vi "Execute.LoadSequences.vi"(8 "error in (no error)":errorcluster, 11 "Cluster":T1={"NIVS.BaseLogPath"=path "", "NIVS.SystemDefinitionFile"=path "", "NIVS.Events"={"SequenceEvent"=refnum, "SystemChangeEvent"=refnum, "WorkspaceEvent"=refnum}, "NIVS.SequenceState"=enum."Idle", "NIVS.GatewayIPAddress"="", "NIVS.DataLogSpecRef"=refnum, "NIVS.DataLogManagerRef"=refnum, "NIVS.LogSessionGUID"="", "NIVS.WorkspaceManager"=refnum, "NIVS.Deployed"=FALSE, "NIVS.ProfileRef"=refnum, "NIVS.ProfileCallback"=refnum, "NIVS.SystemStateRefs"={"CustDatRef"=refnum, "EvtRef"=refnum}, "UI.Abort"=refnum, "UI.Pause"=refnum, "UI.EnableLogging"=refnum, "UI.Start"=refnum, "UI.LogChannels"=refnum, "UI.StartIteration"=refnum, "UI.StartStep"=refnum, "UI.Sequence"=refnum, "UI.PreviewMode"=refnum, "UI.Graph"=refnum, "UI.BaseFileName"=refnum, "UI.Profiles"=refnum, "UI.CurrentStep"=refnum, "UI.CurrentIteration"=refnum, "UI.TotalIterations"=refnum, "Sequence.AbortChannel"="", "Sequence.StepInfoChannel"="", "Sequence.Iterations"=0, "Sequence.IterationInfoChannel"="", "Sequence.#ofColumns"=0, "Events.State"=refnum, "Events.Test Result"=refnum, "Events.Progress"=refnum, "INI.Settings"={"Build Location"=path "C:/Simple Sequence Editor/SequenceRepo", "LoggingLocation"=path ""}}) -> (0 "error out":errorcluster)   [LabVIEW 2013, in "Simple Sequence Tools - Execution.lvlib"]
uses:
  Simple Sequence Tools - Execution.lvlib
  Types/Execuction.StateVariables.ctl
  Types/Execute.UserEventRefs.ctl
  <vilib>/NI Veristand/Execution/Workspace/SystemStateRegEventRef.ctl
  Types/Execution.SequenceState.ctl
  <vilib>/NI Veristand/Execution/DataLogging/DataLoggingSpecification Ref.ctl
  NationalInstruments.VeriStand.ClientAPI
  <vilib>/NI Veristand/Execution/DataLogging/IDataLogging Ref.ctl
  <vilib>/NI Veristand/Execution/Workspace/WorkspaceAPI.ctl
  NationalInstruments.VeriStand.RealTimeSequenceDefinitionApi
  <vilib>/NI Veristand/Execution/Workspace/SystemStateEventRef.ctl
  Shared/Types/INI.Settings
  Shared/Simple Sequence Tools - Shared.lvlib
  <vilib>/NI Veristand/Execution/Workspace/NI_VS Workspace ExecutionAPI.lvlib
  <vilib>/NI Veristand/Execution/DataLogging/NI_VS Data Logging API.lvlib
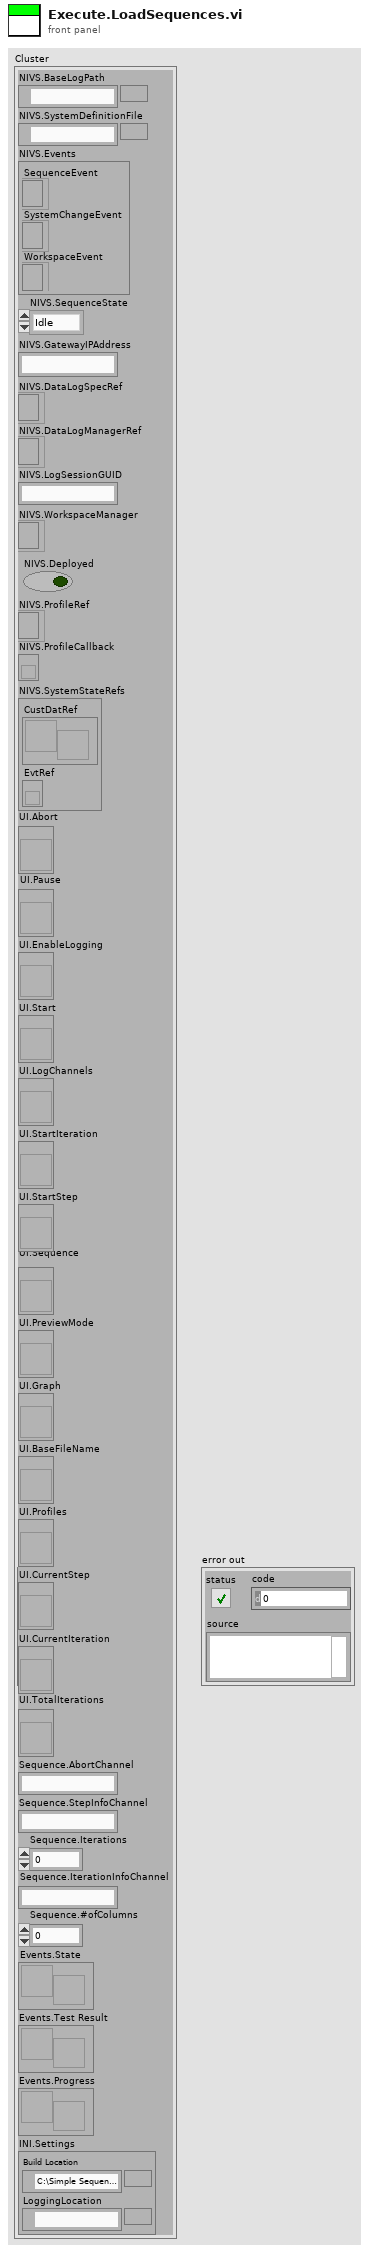
[diagram p1: front panel]
types:
  T1 = typedef "Simple Sequence Tools - Execution.lvlib/Execuction.StateVariables.ctl" = cluster{"NIVS.BaseLogPath":path, "NIVS.SystemDefinitionFile":path, "NIVS.Events":T2, "NIVS.SequenceState":T4, "NIVS.GatewayIPAddress":string, "NIVS.DataLogSpecRef":T5, "NIVS.DataLogManagerRef":T6, "NIVS.LogSessionGUID":string, "NIVS.WorkspaceManager":T7, "NIVS.Deployed":bool, "NIVS.ProfileRef":refnum<k24>, "NIVS.ProfileCallback":refnum<k27>, "NIVS.SystemStateRefs":T8, "UI.Abort":refnum<vi>, "UI.Pause":refnum<vi>, "UI.EnableLogging":refnum<vi>, "UI.Start":refnum<vi>, "UI.LogChannels":refnum<vi>, "UI.StartIteration":refnum<vi>, "UI.StartStep":refnum<vi>, "UI.Sequence":refnum<vi>, "UI.PreviewMode":refnum<vi>, "UI.Graph":refnum<vi>, "UI.BaseFileName":refnum<vi>, "UI.Profiles":refnum<vi>, "UI.CurrentStep":refnum<vi>, "UI.CurrentIteration":refnum<vi>, "UI.TotalIterations":refnum<vi>, "Sequence.AbortChannel":string, "Sequence.StepInfoChannel":string, "Sequence.Iterations":u32, "Sequence.IterationInfoChannel":string, "Sequence.#ofColumns":i32, "Events.State":refnum<user-event>, "Events.Test Result":refnum<user-event>, "Events.Progress":refnum<user-event>, "INI.Settings":T9}
  T2 = typedef "Simple Sequence Tools - Execution.lvlib/Execute.UserEventRefs.ctl" = cluster{"SequenceEvent":refnum<event-registration>, "SystemChangeEvent":T3, "WorkspaceEvent":refnum<event-registration>}
  T3 = typedef "NI_VS Workspace ExecutionAPI.lvlib/SystemStateRegEventRef.ctl" = refnum<event-registration>
  T4 = typedef "Simple Sequence Tools - Execution.lvlib/Execution.SequenceState.ctl" = enum16{"Idle", "Initializing", "Running", "Paused", "Finalizing", "Complete"}
  T5 = typedef "NI_VS Data Logging API.lvlib/DataLoggingSpecification Ref.ctl" = refnum<k24>
  T6 = typedef "NI_VS Data Logging API.lvlib/IDataLogging Ref.ctl" = refnum<k24>
  T7 = typedef "NI_VS Workspace ExecutionAPI.lvlib/WorkspaceAPI.ctl" = refnum<k24>
  T8 = typedef "NI_VS Workspace ExecutionAPI.lvlib/SystemStateEventRef.ctl" = cluster{"CustDatRef":refnum<user-event>, "EvtRef":refnum<k27>}
  T9 = typedef "Simple Sequence Tools - Shared.lvlib/INI.Settings" = cluster{"Build Location":path, "LoggingLocation":path}
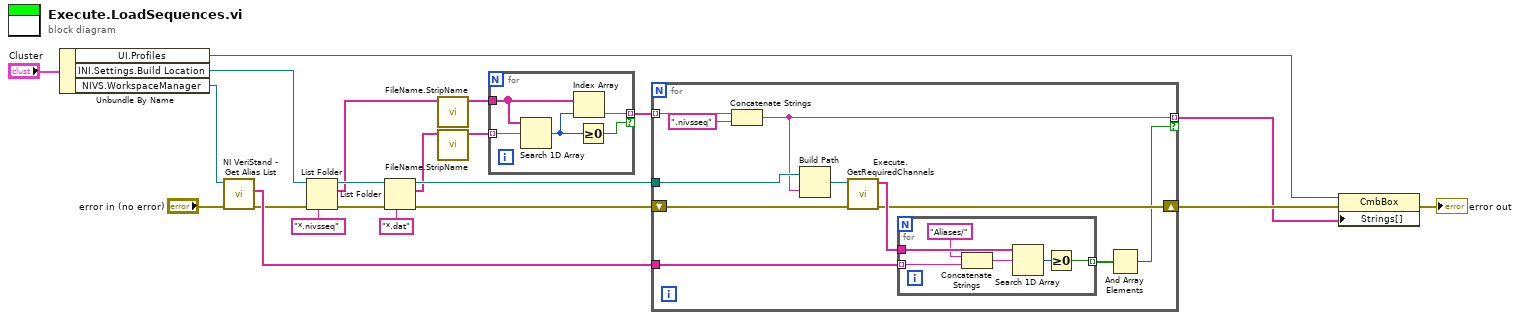
[diagram p0: block diagram]
diagram:
  n1 = Unbundle By Name("Cluster") -> ("UI.Profiles"=w19:refnum<vi>, "INI.Settings.Build Location"=w2:path, "NIVS.WorkspaceManager"=w16:T7)
  n2 = call <vilib>:"NI VeriStand - Get Alias List.vi"("error in (no error)"="error in (no error)", "WorkspaceManager in"=w16) -> ("error out"=w1:errorcluster, "Aliases"=w15:string[])  [unwired: 6 in, 2 out]
  n3 = List Folder(path=w2, pattern="*.nivsseq", error in=w1) -> (path out=w6:path, filenames=w4:string[], error out=w12:errorcluster)  [unwired: 1 in, 1 out]
  n4 = List Folder(path=w6, pattern="*.dat", error in=w12) -> (path out=w13:path, filenames=w5:string[], error out=w14:errorcluster)  [unwired: 1 in, 1 out]
  n5 = call "FileName.StripName.vi"("filenames"=w4) -> ("Array"=w10:string[])  [unwired: 10 in]
  n6 = call "FileName.StripName.vi"("filenames"=w5) -> ("Array"=w9:string[])  [unwired: 10 in]
  n7 = for {
    tunnel: w9 -> [w26] mode=indexing
    tunnel: w10 -> [w25]
    tunnel: [w23] -> w11 mode=indexing if=w22
    n8 = Search 1D Array(1D array=w25, element=w26) -> (index of element=w24:i32)  [unwired: 1 in]
    n9 = Index Array(array=w25, index=w24) -> (element=w23:string)
    n10 = Greater Or Equal To 0?(x=w24) -> (x >= 0?=w22:bool)
  }
  n11 = for {
    tunnel: w11 -> [w37] mode=indexing
    tunnel: w13 -> [w35]
    shift-right: [w29] -> w18
    shift-left: w14 -> [w34]
    tunnel: w15 -> [w31]
    tunnel: [w28] -> w3 mode=indexing if=w27
    n12 = Concatenate Strings(w37, ".nivsseq" ("pattern")) -> (w28:string)
    n13 = Build Path(base path=w35, name or relative path=w28) -> (appended path=w33:path)
    n14 = call "Execute.GetRequiredChannels.vi"("error in (no error)"=w34, "Path"=w33) -> ("error out"=w29:errorcluster, "Channels"=w32:string[])  [unwired: 8 in]
    n15 = for {
      tunnel: w32 -> [w43]
      tunnel: w31 -> [w42] mode=indexing
      tunnel: [w40] -> w30 mode=indexing
      n16 = Concatenate Strings("Aliases/", w42) -> (w39:string)
      n17 = Search 1D Array(1D array=w43, element=w39) -> (index of element=w41:i32)  [unwired: 1 in]
      n18 = Greater Or Equal To 0?(x=w41) -> (x >= 0?=w40:bool)
    }
    n19 = And Array Elements(Boolean array=w30) -> (logical AND=w27:bool)
  }
  n20 = property class="CmbBox"(reference=w19, error in=w18, "Strings[]"=w3) -> (error out=→"error out":errorcluster)  [unwired: 1 out]
